vi "Get Transfer Group Status.vi"(11 "Buffer in":refnum<class "Framework Status.lvclass">) -> (2 "buffer size":refnum<class "Transfer Group Status.lvclass">, 3 "Buffer out":refnum<class "Framework Status.lvclass">)   [LabVIEW 2017, in "DSF Core.lvlib" / "Framework Status.lvclass"]
uses:
  Status/Framework Status.lvclass
  Transfer Group Status/Transfer Group Status.lvclass
  Status/Framework Status.lvclass/Framework Status.ctl
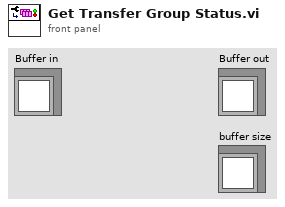
[diagram p1: front panel]
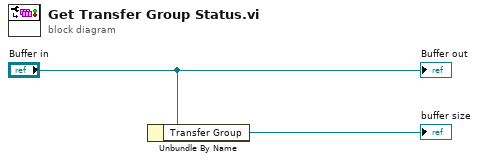
[diagram p0: block diagram]
diagram:
  n1 = Unbundle By Name("Buffer in") -> ("Transfer Group"=→"buffer size":refnum<class "Transfer Group Status.lvclass">)
  "Buffer out" <- "Buffer in"
